vi "Get Base Command.vi"(8 "error in (no error)":errorcluster, 11 "Voltage in":refnum<class "Voltage.lvclass">) -> (0 "error out":errorcluster, 2 "Base Command":string, 3 "Voltage out":refnum<class "Voltage.lvclass">)   [LabVIEW 2023, in "HAF.lvlib" / "Voltage.lvclass"]
doc: "Returns the base command whch is used to build up the overall command string – parameters will be added to this as necessary.  The framework will add the line terminator \\n.\n\nSubclasses MUST override this member and must not add a line terminator on the end of the command; on this class an error is returned."
uses:
  Voltage.lvclass
  Voltage.lvclass/Voltage.ctl
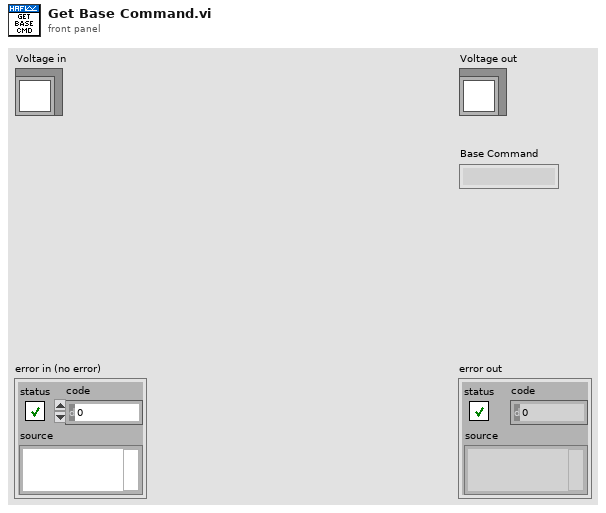
[diagram p1: front panel]
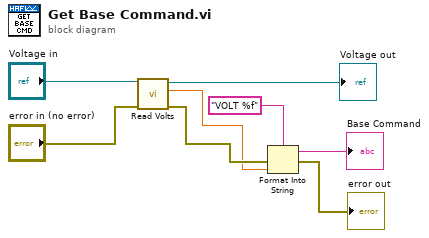
[diagram p0: block diagram]
diagram:
  n1 = call-dynamic "Read Volts.vi"("error in (no error)"="error in (no error)", "Voltage in"="Voltage in") -> ("error out"=w6:errorcluster, "Volts"=w5:dbl, "Voltage out"=→"Voltage out":refnum<class "Voltage.lvclass">)  [unwired: 7 in]
  n2 = Format Into String(format string="VOLT %f", error in=w6, w5) -> (resulting string=→"Base Command":string, error out=→"error out":errorcluster)  [unwired: 1 in]
